vi "Parse and Validate CLI Arguments.vi"(8 "error in":errorcluster, 10 "Custom Parameters":string[](array[string]), 11 "CLI Data in":T1) -> (0 "error out":errorcluster, 3 "CLI Data out":T1)   [LabVIEW 2025]
doc: "This VI comprises the actions to parse CLI arguments and validate correct syntax."
uses:
  Type Definitions/CLI Data--cluster.ctl
  ITSDiscovery/ITSDiscovery.lvclass
  IProcess Executor/IProcess Executor.lvclass
  Type Definitions/Architecture--enum.ctl
  Type Definitions/CLI Argument Setting--cluster.ctl
  <vilib>/Wiresmith Technology/G CLI/Argument Parser/Option Set Class/Option Set.lvclass
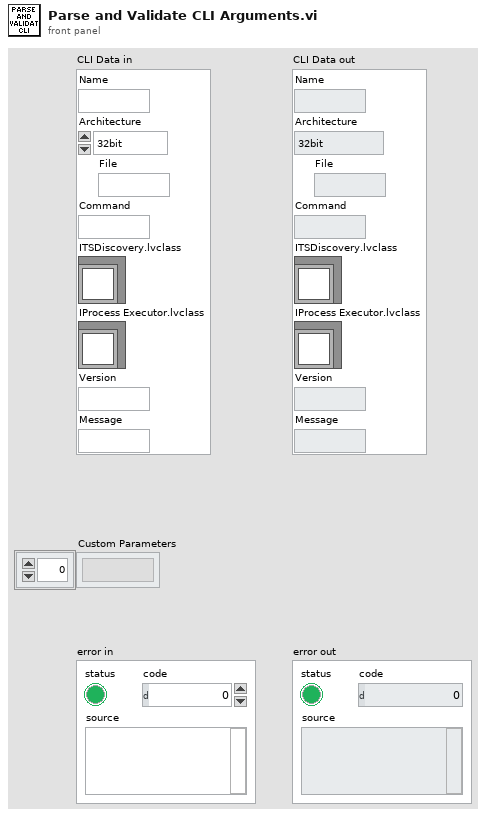
[diagram p1: front panel]
types:
  T1 = typedef "CLI Data--cluster.ctl" = cluster{"Name":string, "Architecture":T2, "File":path, "Command":string, "ITSDiscovery.lvclass":refnum<class "ITSDiscovery.lvclass">, "IProcess Executor.lvclass":refnum<class "IProcess Executor.lvclass">, "Version":string, "Message":string}
  T2 = typedef "Architecture--enum.ctl" = enum16{"32bit", "64bit"}
  T3 = typedef "CLI Argument Setting--cluster.ctl" = cluster{"Name Set":bool, "Version Set":bool, "Architecture Set":bool, "File Set":bool}
  T4 = typedef "Option Parser.lvlib/Option.lvclass/Option Configuration.ctl" = cluster{"Option Type":T5, "Option Labels":string[], "Key":string, "Description":string, "Required":bool, "Default Value":string}
  T5 = typedef "Option Parser.lvlib/Option.lvclass/Argument Type.ctl" = enum16{"flag", "value"}
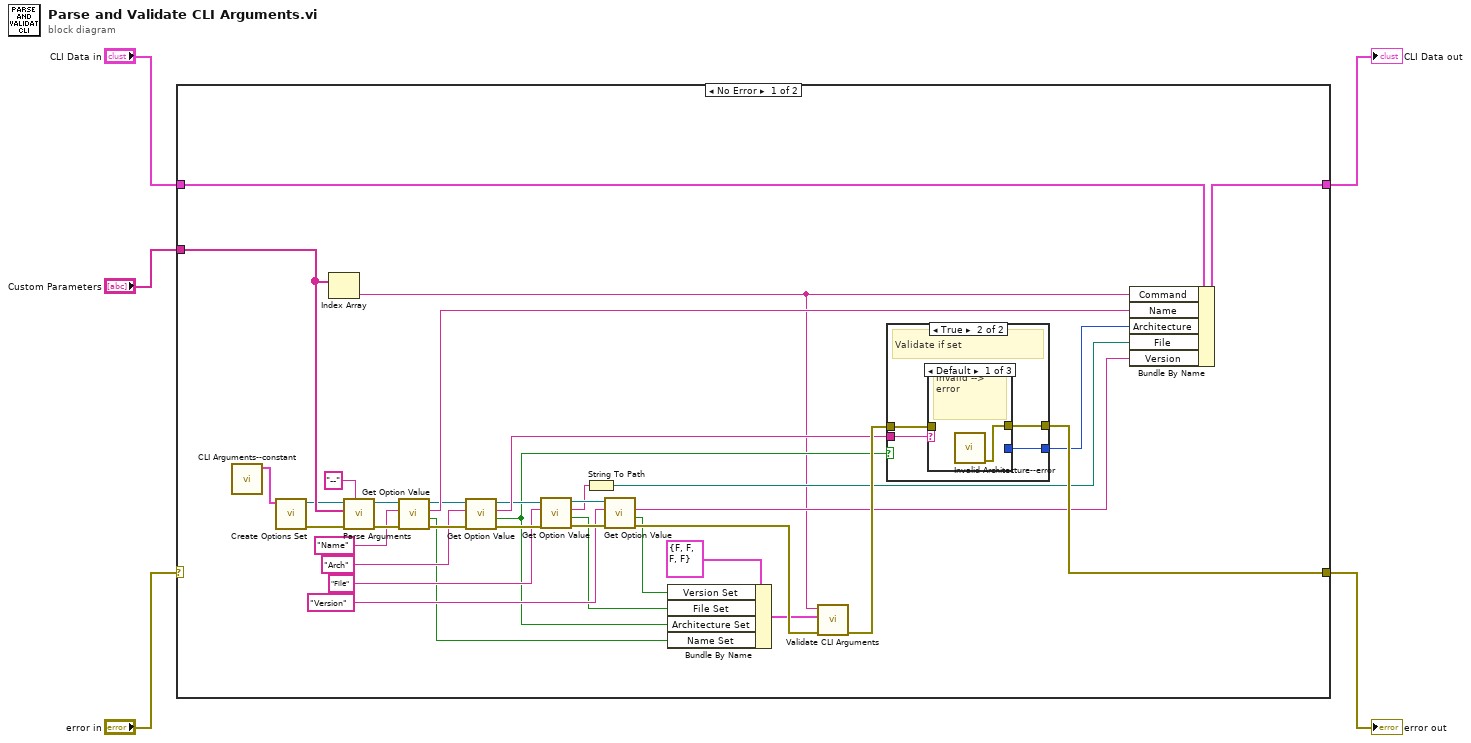
[diagram p0: block diagram]
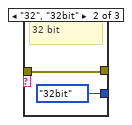
[diagram p3: hidden frame]
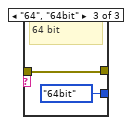
[diagram p4: hidden frame]
diagram:
  n1 = case shown="No Error" "error in" {
    selector: "error in" -> [_ w52]
    tunnel: [w40 w52] -> w5
    tunnel: "Custom Parameters" -> [w23 _]
    tunnel: [w19 w51] -> w2
    tunnel: "CLI Data in" -> [w15 w51]
    frame No Error {
      n2 = call "CLI Arguments--constant.vi"() -> ("Arguments"=w14:T4[])  [unwired: 11 in]
      n3 = call <vilib>:"Create Options Set.vi"("Options"=w14) -> ("error out"=w35:errorcluster, "Option Set out"=w13:refnum<class "Option Set.lvclass">)  [unwired: 9 in]
      n4 = Index Array(array=w23) -> (element=w6:string)  [unwired: 1 in]
      n5 = call <vilib>:"Parse Arguments.vi"("Label Marker (-)"="--", "error in (no error)"=w35, "Arguments"=w23, "Option Set in"=w13) -> ("error out"=w38:errorcluster, "Option Set out"=w26:refnum<class "Option Set.lvclass">)  [unwired: 4 in, 2 out]
      n6 = call <vilib>:"Get Option Value.vi"("error in (no error)"=w38, "Option Key"="Name", "Option Set in"=w26) -> ("error out"=w36:errorcluster, "Set"=w11:bool, "Value"=w20:string, "Option Set out"=w17:refnum<class "Option Set.lvclass">)  [unwired: 5 in]
      n7 = call <vilib>:"Get Option Value.vi"("error in (no error)"=w36, "Option Key"="Arch", "Option Set in"=w17) -> ("error out"=w37:errorcluster, "Set"=w10:bool, "Value"=w30:string, "Option Set out"=w18:refnum<class "Option Set.lvclass">)  [unwired: 5 in]
      n8 = call <vilib>:"Get Option Value.vi"("error in (no error)"=w37, "Option Key"="File", "Option Set in"=w18) -> ("error out"=w39:errorcluster, "Set"=w9:bool, "Value"=w21:string, "Option Set out"=w29:refnum<class "Option Set.lvclass">)  [unwired: 5 in]
      n9 = String To Path(string=w21) -> (path=w22:path)
      n10 = call <vilib>:"Get Option Value.vi"("error in (no error)"=w39, "Option Key"="Version", "Option Set in"=w29) -> ("error out"=w34:errorcluster, "Set"=w8:bool, "Value"=w32:string)  [unwired: 5 in, 1 out]
      n11 = Bundle By Name(cluster=T3 {"Name Set"=FALSE, "Version Set"=FALSE, "Architecture Set"=FALSE, "File Set"=FALSE} ("CLI Arguments Setting"), "Version Set"=w8, "File Set"=w9, "Architecture Set"=w10, "Name Set"=w11) -> (w7:T3)
      n12 = call "Validate CLI Arguments.vi"("error in"=w34, "CLI Arguments Setting"=w7, "Command"=w6) -> ("error out"=w33:errorcluster)  [unwired: 8 in]
      n13 = case shown="True" w10 {
        tunnel: w30 -> [_ w43]
        tunnel: [_ w42] -> w31
        tunnel: w33 -> [w41 w45]
        tunnel: [w41 w44] -> w40
        frame False {
          # "Not set."
        }
        frame True {
          # "Validate if set"
          n14 = case shown="Default" w43 {
            tunnel: [_ Architecture--enum."32bit" ("Architecture") Architecture--enum."64bit" ("Architecture")] -> w42
            tunnel: w45 -> [_ w48 w50]
            tunnel: [w46 w48 w50] -> w44
            frame Default {
              # "Invalid --> error"
              n15 = call "Invalid Architecture--error.vi"() -> ("error out"=w46:errorcluster)  [unwired: 11 in]
            }
            frame "32", "32bit" {
              # "32 bit"
            }
            frame "64", "64bit" {
              # "64 bit"
            }
          }
        }
      }
      n16 = Bundle By Name(cluster=w15, "Command"=w6, "Name"=w20, "Architecture"=w31, "File"=w22, "Version"=w32) -> (w19:T1)
    }
    frame Error {
      # "Pass error without further action"
    }
  }
  "error out" <- w5
  "CLI Data out" <- w2
